vi "GenNewTraj.vi"(8 "Stoopid Overlap %":dbl min=0.0, 9 "Velocities":dbl[](array[numeric]), 10 "Parameters":T2={"Sample Period (s)"=0.0, "Limits"={"Velocity (fps)"=6.0, "Accel (fps^2)"=15.0, "Jerk (fps^3)"=150.0, "StoopidFast (fps)"=6.0}, "Conditions"={"vInitial (fps)"=0.0, "vFinal (fps)"=0.0}, "output cluster"={"Angular \nAccelerations"=[], "Override Limits?"=[]}} {"Limits"."StoopidFast (fps)" min=0.0; "Limits"."Jerk (fps^3)" min=0.0 step=1.0; "Limits"."Accel (fps^2)" min=0.0; "Limits"."Velocity (fps)" min=0.0}, 11 "Points in":cluster{"x":dbl, "y":dbl, "th":dbl}[](array[cluster])) -> (0 "Time (s)":dbl, 1 "Valid":bool, 2 "Trajectory Data":T3(array[cluster]), 3 "Updated Waypoints":cluster{"x":dbl, "y":dbl, "th":dbl}[](array[cluster]), 4 "Distance (ft)":dbl)   [LabVIEW 2019]
uses:
  Limits.ctl
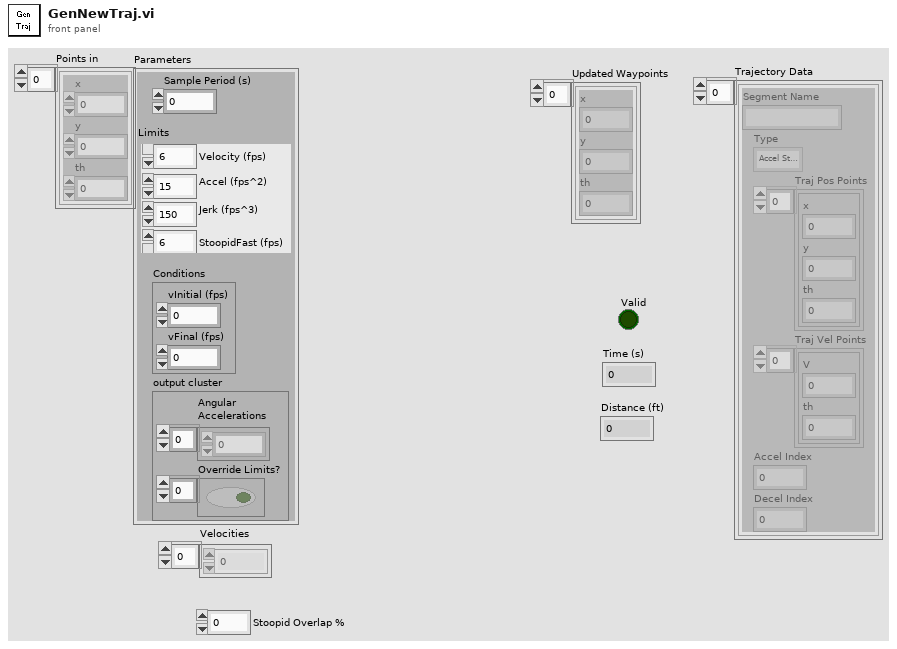
[diagram p1: front panel]
types:
  T1 = typedef "Limits.ctl" = cluster{"Velocity (fps)":dbl, "Accel (fps^2)":dbl, "Jerk (fps^3)":dbl, "StoopidFast (fps)":dbl}
  T2 = cluster{"Sample Period (s)":dbl, "Limits":T1, "Conditions":cluster{"vInitial (fps)":dbl, "vFinal (fps)":dbl}, "output cluster":cluster{"Angular \nAccelerations":dbl[], "Override Limits?":bool[]}}
  T3 = cluster{"Segment Name":string, "Type":enum16{"Accel Straight", "Const Straight", "Blend", "Circle"}, "Traj Pos Points":cluster{"x":dbl, "y":dbl, "th":dbl}[], "Traj Vel Points":cluster{"V":dbl, "th":dbl}[], "Accel Index":i32, "Decel Index":i32}[]
  T4 = cluster{"vInitial (fps)":dbl, "vFinal (fps)":dbl}
  T5 = cluster{"Angular \nAccelerations":dbl[], "Override Limits?":bool[]}
  T6 = cluster{"output cluster":cluster{"Angular \nAccelerations":dbl[], "Override Limits?":bool[]}, "Velocities":dbl[]}
  T7 = cluster{"Trajectory Data":cluster{"Segment Name":string, "Type":enum16{"Accel Straight", "Const Straight", "Blend", "Circle"}, "Traj Pos Points":cluster{"x":dbl, "y":dbl, "th":dbl}[], "Traj Vel Points":cluster{"V":dbl, "th":dbl}[], "Accel Index":i32, "Decel Index":i32}[], "Time (s)":dbl, "Valid":bool, "Updated Waypoints":cluster{"x":dbl, "y":dbl, "th":dbl}[], "Distance (ft)":dbl}
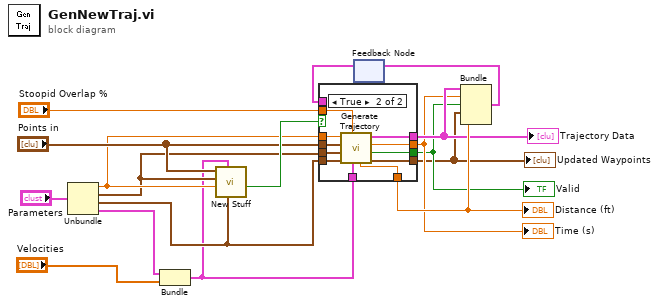
[diagram p0: block diagram]
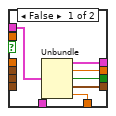
[diagram p2: hidden frame]
diagram:
  n1 = Unbundle("Parameters") -> ("Sample Period (s)"=w7:dbl, "Limits"=w6:T1, "Conditions"=w5:T4, "output cluster"=w3:T5)
  n2 = Bundle("output cluster"=w3, "Velocities"="Velocities") -> (w2:T6)  [unwired: 1 in]
  n3 = call "New Stuff.vi"("Conditions"=w5, "Overrides"=w2, "Sample Period (s)"=w7, "Limits"=w6, "Points in"="Points in") -> ("result"=w17:bool)  [unwired: 6 in]
  n4 = feedback #1() -> (w14:T7)  [unwired: 1 in]
  n5 = case shown="True" w17 {
    tunnel: [w20 w34] -> w10
    tunnel: [w21 w33] -> w11
    tunnel: [w18 w32] -> w16
    tunnel: w5 -> [_ w31]
    tunnel: w6 -> [_ w30]
    tunnel: w2 -> [_ w29]
    tunnel: "Points in" -> [_ w28]
    tunnel: [w19 w27] -> w9
    tunnel: [w22 w26] -> w12
    tunnel: w7 -> [_ w25]
    tunnel: w14 -> [w23 _]
    tunnel: "Stoopid Overlap %" -> [_ w24]
    frame False {
      n6 = Unbundle(w23) -> ("Trajectory Data"=w22:T3, "Time (s)"=w21:dbl, "Valid"=w20:bool, "Updated Waypoints"=w19:cluster{"x":dbl, "y":dbl, "th":dbl}[], "Distance (ft)"=w18:dbl)
    }
    frame True {
      n7 = call "Generate Trajectory.vi"("Overrides"=w29, "Stoopid Overlap %"=w24, "Conditions"=w31, "Limits"=w30, "WayPoints"=w28, "Sample Period (s)"=w25) -> ("Updated Waypoints"=w27:cluster{"x":dbl, "y":dbl, "th":dbl}[], "Valid"=w34:bool, "Time (s)"=w33:dbl, "Trajectory Data"=w26:T3, "Distance (ft)"=w32:dbl)  [unwired: 1 in]
    }
  }
  "Distance (ft)" <- w16
  "Trajectory Data" <- w12
  "Time (s)" <- w11
  "Valid" <- w10
  "Updated Waypoints" <- w9
  n8 = Bundle("Trajectory Data"=w12, "Time (s)"=w11, "Valid"=w10, "Updated Waypoints"=w9, "Distance (ft)"=w16) -> (w13:T7)  [unwired: 1 in]
  n9 = feedback-in #1(w13) -> ()
